vi "Teleop_System_Execute.vi"(11 "Teleop Elapsed Seconds":dbl) -> ()   [LabVIEW 2019]
uses:
  <vilib>/Rock Robotics/WPI/Joystick/XBox Axes Indexer.ctl
  <vilib>/Rock Robotics/WPI/Joystick/XBox Buttons Indexer.ctl
  <vilib>/Rock Robotics/WPI/ThirdParty/JAS_Junk/TrajLib/VI/Util_GetTime_U32.vi
  <vilib>/Rock Robotics/WPI/ThirdParty/JAS_Junk/TrajLib/VI/numCmd_Send_Generic.vi
  <vilib>/Rock Robotics/WPI/ThirdParty/JAS_Junk/TrajLib/VI/numCmd_ObtainQueue_Generic.vi
  <vilib>/Rock Robotics/WPI/ThirdParty/JAS_Junk/TrajLib/VI/Util_GetTime_U64.vi
  Swerve_Drive_System/SWERVE_DRIVE_GLOBALS.vi
  <vilib>/Rock Robotics/WPI/Utilities/WPI_GetSetVariantRefNum.vi
  <vilib>/Rock Robotics/Network Tables/NT Write Numeric Array.vi
  <vilib>/Rock Robotics/Network Tables/NT Write Boolean Array.vi
  Sweve_Trajectory_Following/SDO_TRAJECTORY_GLOBALS.vi
  <vilib>/Rock Robotics/WPI/ThirdParty/JAS_Junk/TrajLib/Trajectory_Library.lvlib
  <vilib>/Rock Robotics/Network Tables/NT Write Integer Array.vi
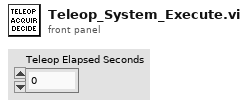
[diagram p1: front panel]
types:
  T1 = typedef "XBox Axes Indexer.ctl" = enum16{"Left X", "Left Y", "Left Trigger", "Right Trigger", "Right X", "Right Y"}
  T2 = typedef "XBox Buttons Indexer.ctl" = enum16{"A", "B", "X", "Y", "Left Bumper", "Right Bumper", "Back", "Start", "Left Joystick", "Right Joystick"}
  T3 = typedef "WPI_JoystickDevRef.ctl" = cluster{"Device":T4}
  T4 = typedef "WPI_JoystickDeviceEnum.ctl" = enum16{"USB 0", "USB 1", "USB 2", "USB 3", "USB 4", "USB 5"}
  T5 = typedef "Trajectory_Library.lvlib/CHASSIS_SPEEDS.ctl" = cluster{"vX":dbl, "vY":dbl, "vOmega":dbl}
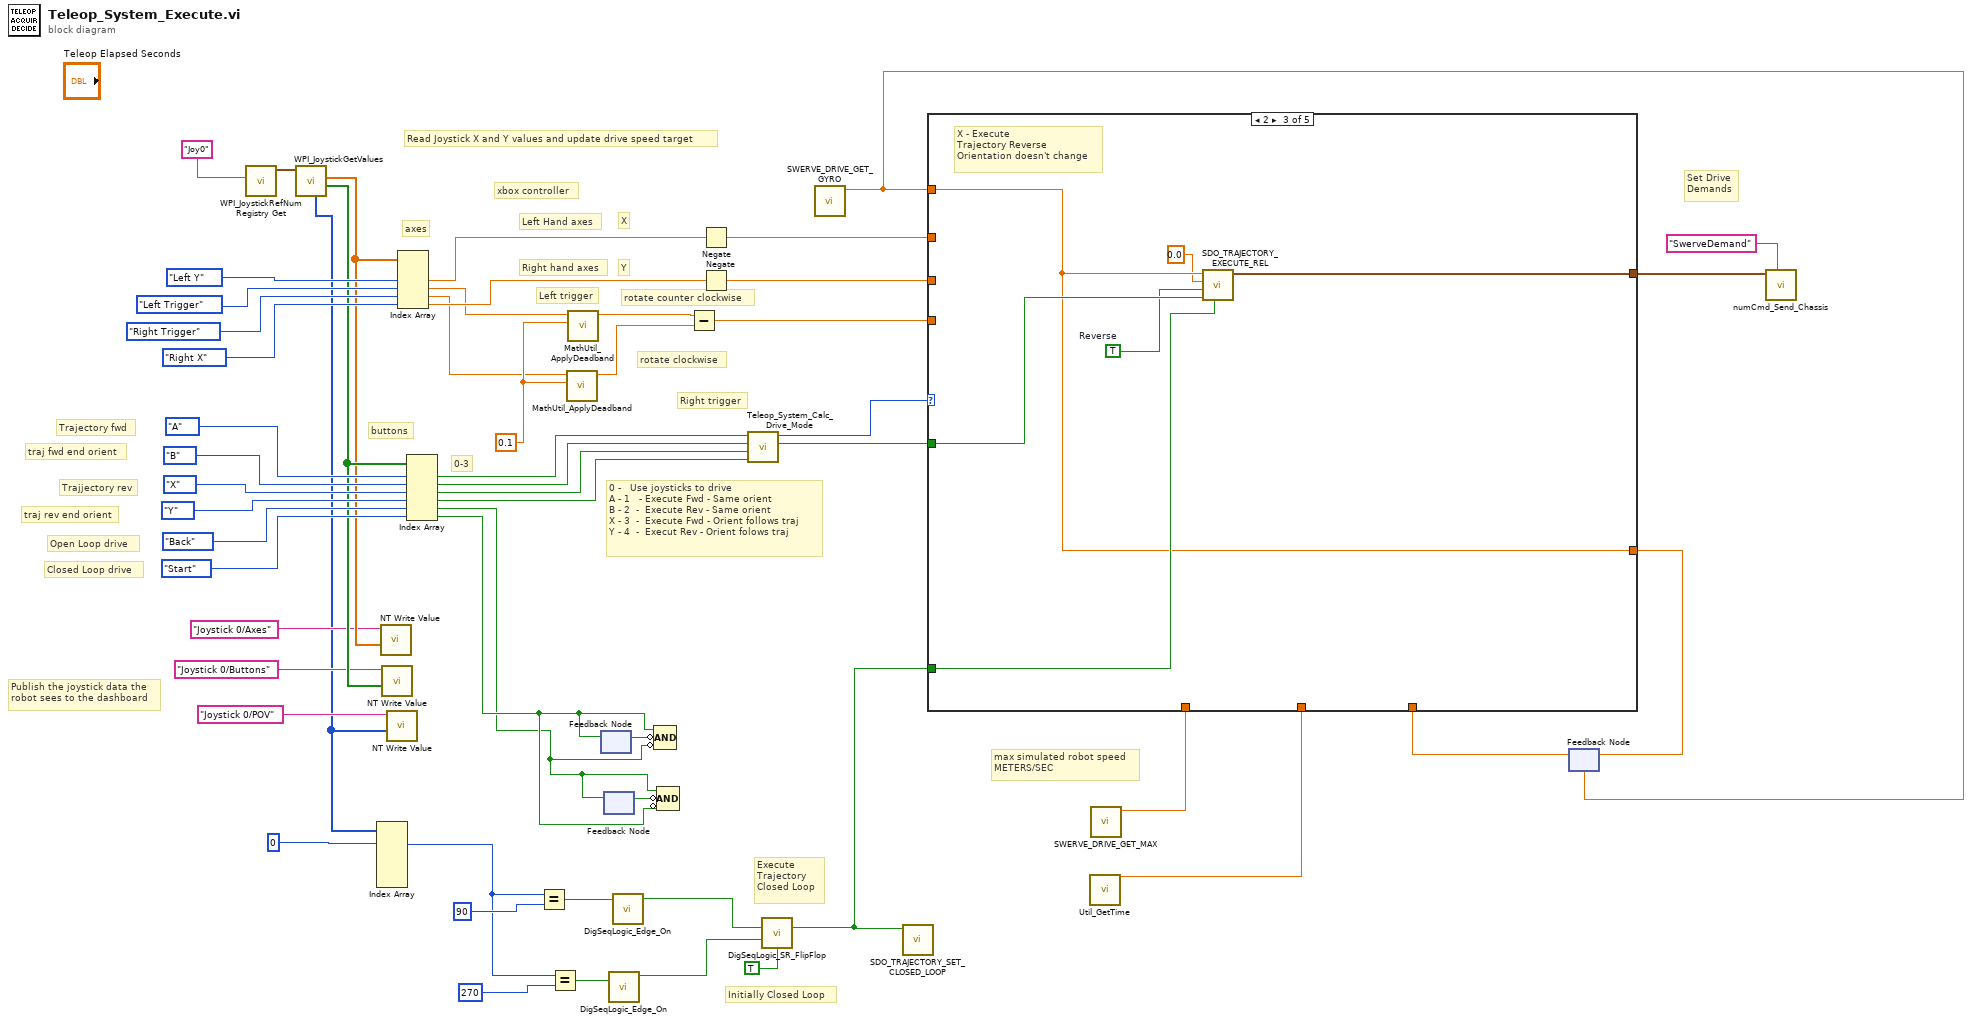
[diagram p0: block diagram]
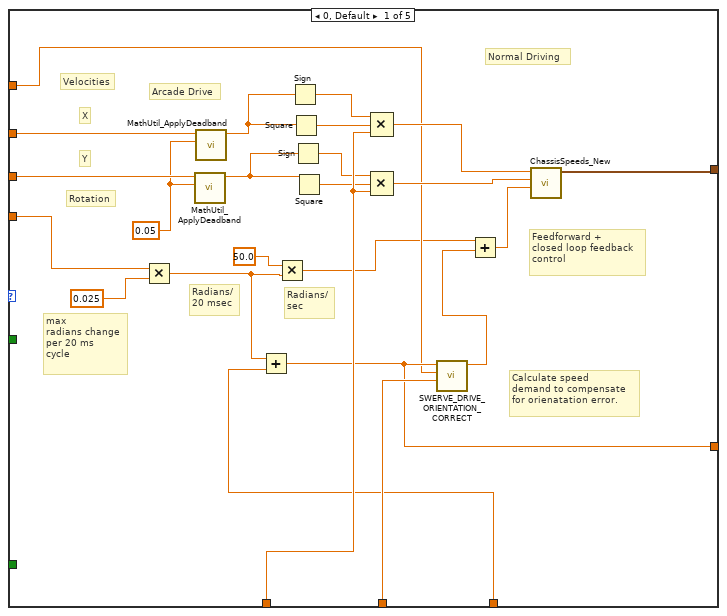
[diagram p2: hidden frame]
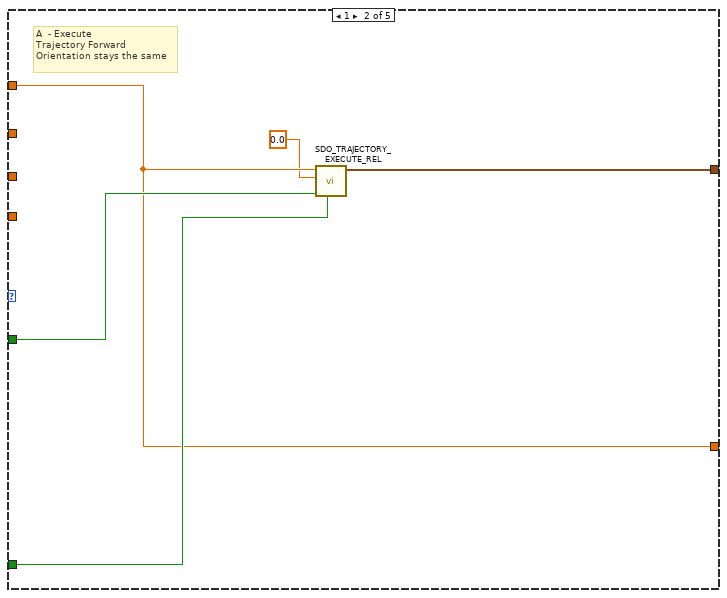
[diagram p3: hidden frame]
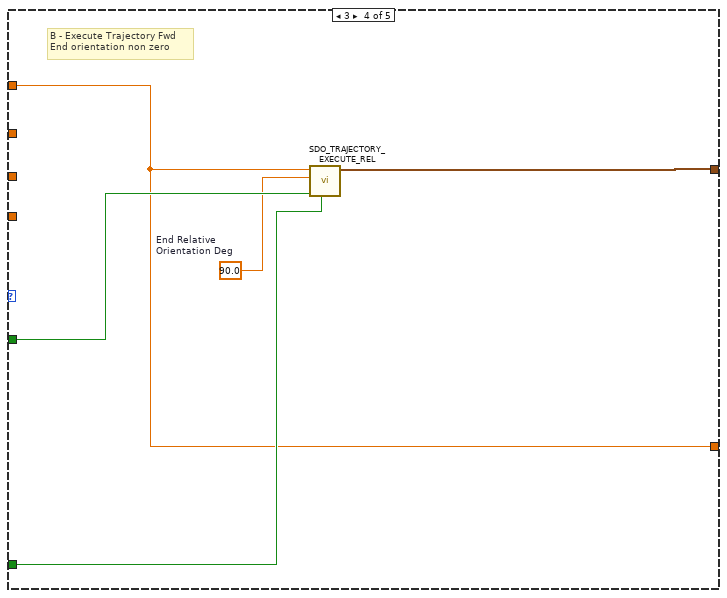
[diagram p4: hidden frame]
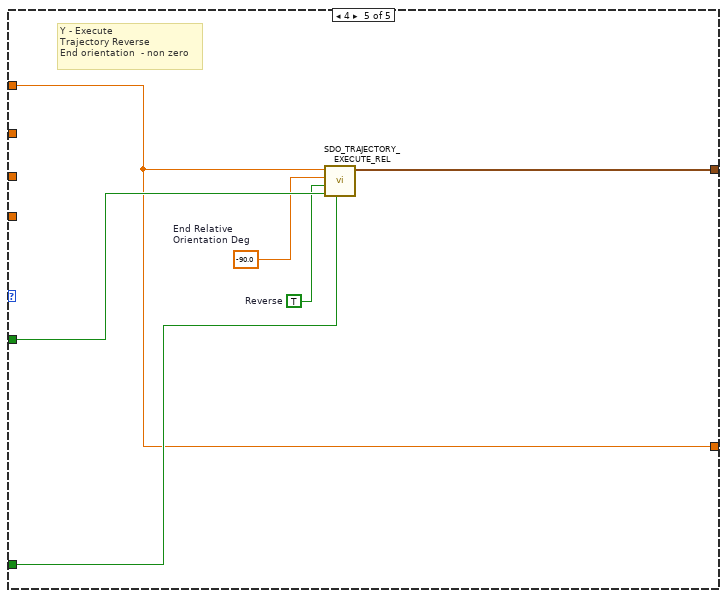
[diagram p5: hidden frame]
diagram:
  w42 = 0.1 ("Deadband")
  # "traj rev end orient"
  # "traj fwd end orient"
  # "Trajjectory rev"
  # "Closed Loop drive"
  # "Open Loop drive"
  # "Trajectory fwd"
  # "0 -   Use joysticks to drive\nA - 1   - Execute Fwd - Same orient\nB - 2  -  Execute Rev - Same orient\nX - 3  -  Execute Fwd - Orient follows traj\nY - 4  -  Execut Rev - Orient folows traj"
  # "Execute\nTrajectory\nClosed Loop"
  # "Set Drive\nDemands"
  # "Initially Closed Loop"
  # "0-3"
  # "xbox controller"
  # "Left trigger"
  # "rotate counter clockwise"
  # "Right trigger"
  # "rotate clockwise"
  # "Left Hand axes"
  # "Right hand axes"
  # "Y"
  # "X"
  # "buttons"
  # "axes"
  # "max simulated robot speed\nMETERS/SEC"
  # "Publish the joystick data the\nrobot sees to the dashboard"
  # "Read Joystick X and Y values and update drive speed target"
  n1 = call <vilib>:"WPI_JoystickRefNum Registry Get.vi"("refnum name"="Joy0") -> ("JoystickDevRef"=w22:T3)  [unwired: 1 in, 9 out]
  n2 = call <vilib>:"WPI_JoystickGetValues.vi"("JoystickDevRef"=w22) -> ("Buttons"=w26:bool[], "Axes"=w25:dbl[], "POVs"=w9:i16[])  [unwired: 6 in, 2 out]
  n3 = Index Array(array=w9, index #1=0 ("index")) -> (element #1=w5:i16)  [unwired: 5 in, 5 out]
  n4 = call-poly <vilib>:"NT Write Value.vi"("value"=w25, "name"="Joystick 0/Axes" ("Name")) -> ()  [unwired: 9 in, 1 out]
  n5 = call-poly <vilib>:"NT Write Value.vi"("value"=w26, "name"="Joystick 0/Buttons" ("Name")) -> ()  [unwired: 9 in, 1 out]
  n6 = call-poly <vilib>:"NT Write Value.vi"("value"=w9, "name"="Joystick 0/POV" ("Name")) -> ()  [unwired: 9 in, 1 out]
  n7 = Index Array(array=w25, index #2=XBox_Axes_Indexer."Left Y" ("XBox Axes"), index #3=XBox_Axes_Indexer."Left Trigger" ("XBox Axes"), index #4=XBox_Axes_Indexer."Right Trigger" ("XBox Axes"), index #5=XBox_Axes_Indexer."Right X" ("XBox Axes")) -> (element #2=w34:dbl, element #3=w16:dbl, element #4=w14:dbl, element #5=w35:dbl)  [unwired: 1 in, 1 out]
  n8 = Index Array(array=w26, index #1=XBox_Buttons_Indexer."A" ("XBox Buttons"), index #2=XBox_Buttons_Indexer."B" ("XBox Buttons"), index #3=XBox_Buttons_Indexer."X" ("XBox Buttons"), index #4=XBox_Buttons_Indexer."Y" ("XBox Buttons"), index #5=XBox_Buttons_Indexer."Back" ("XBox Buttons"), index #6=XBox_Buttons_Indexer."Start" ("XBox Buttons")) -> (element #1=w27:bool, element #2=w36:bool, element #3=w37:bool, element #4=w51:bool, element #5=w40:bool, element #6=w41:bool)
  n9 = Equal?(x=w5, y=i16 90) -> (x = y?=w4:bool)
  n10 = Equal?(x=w5, y=i16 270) -> (x = y?=w3:bool)
  n11 = call <vilib>:"MathUtil_ApplyDeadband.vi"("Deadband"=w42, "Value"=w14) -> ("Result"=w13:dbl)  [unwired: 9 in]
  n12 = call <vilib>:"MathUtil_ApplyDeadband.vi"("Deadband"=w42, "Value"=w16) -> ("Result"=w15:dbl)  [unwired: 9 in]
  n13 = feedback #1() -> (w38:bool)  [unwired: 1 in]
  n14 = feedback-in #1(w41) -> ()
  n15 = feedback #2() -> (w39:bool)  [unwired: 1 in]
  n16 = feedback-in #2(w40) -> ()
  n17 = call <vilib>:"DigSeqLogic_Edge_On.vi"("Input"=w3) -> ("On Edge"=w1:bool)  [unwired: 10 in]
  n18 = call <vilib>:"DigSeqLogic_Edge_On.vi"("Input"=w4) -> ("On Edge"=w2:bool)  [unwired: 10 in]
  n19 = Compound Arithmetic op=AND(w41, invert w38, invert w40) -> ()  [unwired: 1 out]
  n20 = Compound Arithmetic op=AND(w40, invert w39, invert w41) -> ()  [unwired: 1 out]
  n21 = Subtract(x=w15, y=w13) -> (x-y=w31:dbl)
  n22 = Negate(x=w34) -> (-x=w32:dbl)
  n23 = Negate(x=w35) -> (-x=w33:dbl)
  n24 = call "Teleop_System_Calc_Drive_Mode.vi"("Traj Rev Follow Orient"=w51, "Traj Rev Same Orient"=w37, "Traj Fwd Follow Orient"=w36, "Traj Fwd Same Orient"=w27) -> ("Dirve Mode Changed"=w29:bool, "Drive Mode"=w28:i32)  [unwired: 6 in]
  n25 = call <vilib>:"DigSeqLogic_SR_FlipFlop.vi"("Set"=w2, "Reset"=w1, "Initial Value"=TRUE) -> ("Output"=w44:bool)  [unwired: 11 in, 1 out]
  n26 = call "SWERVE_DRIVE_GET_GYRO.vi"() -> ("Gyro Heading Radians"=w18:dbl)  [unwired: 11 in]
  n27 = call "SDO_TRAJECTORY_SET_CLOSED_LOOP.vi"("AUTO_CLOSED_LOOP"=w44) -> ()  [unwired: 11 in]
  n28 = call <vilib>:"Util_GetTime.vi"() -> ("FPGA_Time_Seconds"=w20:dbl)  [unwired: 9 in, 2 out]
  n29 = call "SWERVE_DRIVE_GET_MAX.vi"() -> ("Max Wheel Vel (Meter/Sec)"=w30:dbl)  [unwired: 10 in, 1 out]
  n30 = feedback #3(w18) -> (w17:dbl)
  n31 = case shown="2" w28 {
    tunnel: w33 -> [w69 _ _ _ _]
    tunnel: w30 -> [w79 _ _ _ _]
    tunnel: w29 -> [_ w84 w90 w95 w101]
    tunnel: w32 -> [w71 _ _ _ _]
    tunnel: w31 -> [w73 _ _ _ _]
    tunnel: w18 -> [w62 w81 w86 w92 w98]
    tunnel: w44 -> [_ w83 w88 w94 w100]
    tunnel: [w65 w82 w87 w93 w99] -> w12
    tunnel: w20 -> [w64 _ _ _ _]
    tunnel: [w63 w81 w86 w92 w98] -> w19
    tunnel: w17 -> [w61 _ _ _ _]
    frame 0, Default {
      w68 = 0.05 ("Deadband")
      # "Feedforward +\nclosed loop feedback\ncontrol"
      # "Radians/\nsec"
      # "Radians/\n20 msec"
      # "Calculate speed\ndemand to compensate\nfor orienatation error."
      # "Normal Driving"
      # "Velocities"
      # "Rotation"
      # "max \nradians change\nper 20 ms\ncycle"
      # "Y"
      # "X"
      # "Arcade Drive"
      n32 = Multiply(x=w73, y=0.025) -> (x*y=w60:dbl)
      n33 = call <vilib>:"MathUtil_ApplyDeadband.vi"("Deadband"=w68, "Value"=w69) -> ("Result"=w72:dbl)  [unwired: 9 in]
      n34 = call <vilib>:"MathUtil_ApplyDeadband.vi"("Deadband"=w68, "Value"=w71) -> ("Result"=w70:dbl)  [unwired: 9 in]
      n35 = Add(x=w60, y=w61) -> (x+y=w63:dbl)
      n36 = Multiply(x=50.0, y=w60) -> (x*y=w57:dbl)
      n37 = Sign(1:w70) -> (0:w77:dbl)
      n38 = Square(x=w70) -> (x^2=w78:dbl)
      n39 = Sign(1:w72) -> (0:w75:dbl)
      n40 = Square(x=w72) -> (x^2=w76:dbl)
      n41 = Compound Arithmetic op=MULTIPLY(w77, w78, w79) -> (w67:dbl)
      n42 = Compound Arithmetic op=MULTIPLY(w75, w76, w79) -> (w66:dbl)
      n43 = call "SWERVE_DRIVE_ORIENTATION_CORRECT.vi"("FPGA_Time_Seconds"=w64, "Gyro Heading Radians"=w62, "Drv Rotation Orentation Dmd  Radians"=w63) -> ("CO-ControlOutput"=w56:dbl)  [unwired: 8 in]
      n44 = Add(x=w57, y=w56) -> (x+y=w58:dbl)
      n45 = call <vilib>:"ChassisSpeeds_New.vi"("vAngular"=w58, "vY"=w66, "vX"=w67) -> ("CHASSIS"=w65:T5)  [unwired: 8 in]
    }
    frame 1 {
      # "A  - Execute\nTrajectory Forward\nOrientation stays the same"
      n46 = call "SDO_TRAJECTORY_EXECUTE_REL.vi"("EnableClosedLoop"=w83, "Init"=w84, "End Relative\nOrientation Deg"=0.0 ("End Relative\nOrientation Deg"), "Gyro Heading\nRAD"=w81) -> ("Chassis Velocity Target"=w82:T5)  [unwired: 6 in, 1 out]
    }
    frame 2 {
      w89 = TRUE  # Reverse
      # "X - Execute \nTrajectory Reverse\nOrientation doesn't change"
      n47 = call "SDO_TRAJECTORY_EXECUTE_REL.vi"("EnableClosedLoop"=w88, "Init"=w90, "Reverse"=w89, "End Relative\nOrientation Deg"=0.0 ("End Relative\nOrientation Deg"), "Gyro Heading\nRAD"=w86) -> ("Chassis Velocity Target"=w87:T5)  [unwired: 5 in, 1 out]
    }
    frame 3 {
      w91 = 90.0  # End Relative Orientation Deg
      # "B - Execute Trajectory Fwd \nEnd orientation non zero"
      n48 = call "SDO_TRAJECTORY_EXECUTE_REL.vi"("EnableClosedLoop"=w94, "Init"=w95, "End Relative\nOrientation Deg"=w91, "Gyro Heading\nRAD"=w92) -> ("Chassis Velocity Target"=w93:T5)  [unwired: 6 in, 1 out]
    }
    frame 4 {
      w96 = -90.0  # End Relative Orientation Deg
      w97 = TRUE  # Reverse
      # "Y - Execute\nTrajectory Reverse\nEnd orientation  - non zero"
      n49 = call "SDO_TRAJECTORY_EXECUTE_REL.vi"("EnableClosedLoop"=w100, "Init"=w101, "Reverse"=w97, "End Relative\nOrientation Deg"=w96, "Gyro Heading\nRAD"=w98) -> ("Chassis Velocity Target"=w99:T5)  [unwired: 5 in, 1 out]
    }
  }
  n50 = feedback-in #3(w19) -> ()
  n51 = call <vilib>:"numCmd_Send_Chassis.vi"("Command Name"="SwerveDemand", "Chassis Speeds"=w12) -> ()  [unwired: 9 in, 1 out]
